vi "forced_vibration_and_shock.vi"() -> ()   [LabVIEW 2024]
uses:
  <vilib>/DAQmx/read.llb/DAQmx Read (Analog 1D Wfm NChan NSamp).vi
  <vilib>/DAQmx/create/channels.llb/DAQmx Create Channel (AI-Voltage-Basic).vi
  <vilib>/DAQmx/create/channels.llb/DAQmx Create Channel (AI-Acceleration-Accelerometer).vi
  <vilib>/DAQmx/configure/timing.llb/DAQmx Timing (Sample Clock).vi
  <vilib>/express/express analysis/Spectral/Block/exnSpectralBlock spectral measurements RMS poly.vi
  <vilib>/express/express analysis/Spectral/Block/exnSpectralBlock spectral measurements RMS WFM.vi
  <vilib>/express/express shared/transition.llb/Dynamic To Waveform Array.vi
  <vilib>/express/express signal manip/GetorSetDDTAttributes/Set DDT Attributes/SetT0.vi
  <vilib>/express/express shared/transition.llb/Waveform Array To Dynamic.vi
  <vilib>/DAQmx/miscellaneous.llb/DAQmx Fill In Error Info.vi
  <vilib>/express/express analysis/Spectral/Block/exnSpectralBlock spectral measurements RMS DDT.vi
  <vilib>/express/express analysis/Spectral/XNode/ExpressSpectralMeasurementsBlockNode.xnode
  <vilib>/express/express signal manip/GetorSetDDTAttributes/Set DDT Attributes/Set DDT Properties.xnode
  <resource>/objmgr/daqmx.rc
  <vilib>/measure/NI_MAPro.lvlib
panel:
  out "Waveform Graph 6":waveform(dbl)(graph)
  out "error out 4":errorcluster
  in  "error in (no error) 4":errorcluster
  in  "sampling info 3":cluster{"Fs":dbl, "#s":dbl}={"Fs"=1000.0, "#s"=1000.0} {"Fs" format="%.2p"}
  in  "frequency 3":dbl=10.0 format="%0.2p"
  in  "amplitude 3":dbl=1.0 format="%0.2p"
  in  "formula 3":string="sin(w*t)*sin(2*pi(1)*t)"
  out "Waveform Graph 5":waveform(dbl)(graph)
  out "Array":dbl[](array[numeric])
  in  "Numeric 2":dbl
  in  "Numeric 3":dbl
  in  "?":path
  out "Filename Out 3":path caption="Filename Out"
  out "AO_output_acc":waveform(dbl)(graph)
  out "AO_input_acc":waveform(dbl)(graph)
  out "AO_Voltage":waveform(dbl)(graph)
  out "FFT magnitude 3":dynamicdata(graph)
  out "ACC Time domain 3":dynamicdata(graph)
  out "VOLT Time domain 2":dynamicdata(graph)
  out "FFT magnitude 2":dynamicdata(graph)
  out "error out 2":errorcluster
  in  "error in (no error) 2":errorcluster
  in  "sampling info 2":cluster{"Fs":dbl, "#s":dbl}={"Fs"=1000.0, "#s"=1000.0} {"Fs" format="%.2p"}
  in  "frequency 2":dbl=10.0 format="%0.2p"
  in  "amplitude 2":dbl=1.0 format="%0.2p"
  in  "formula 2":string="sin(w*t)*sin(2*pi(1)*t)"
  out "Waveform Graph 4":waveform(dbl)(graph)
  out "error out":errorcluster
  in  "error in (no error)":errorcluster
  in  "sampling info":cluster{"Fs":dbl, "#s":dbl}={"Fs"=1000.0, "#s"=1000.0} {"Fs" format="%.2p"}
  in  "frequency":dbl=10.0 format="%0.2p"
  in  "amplitude":dbl=1.0 format="%0.2p"
  in  "formula":string="sin(w*t)*sin(2*pi(1)*t)"
  out "Waveform Graph 3":waveform(dbl)(graph)
  out "end index":i32
  out "start index":i32
  in  "end time":dbl
  in  "start time":dbl
  out "FFT excitation":cluster{"f0":dbl, "df":dbl, "magnitude":dbl[]}(graph)
  in  "voltage scale":dbl
  in  "output frequency":dbl
  # "frame_1"
  # "frame_3"
  # "0.1*sin(2*3.1416*5*t) + 2*exp(-((t-4)^2)/(2*0.05^2))"
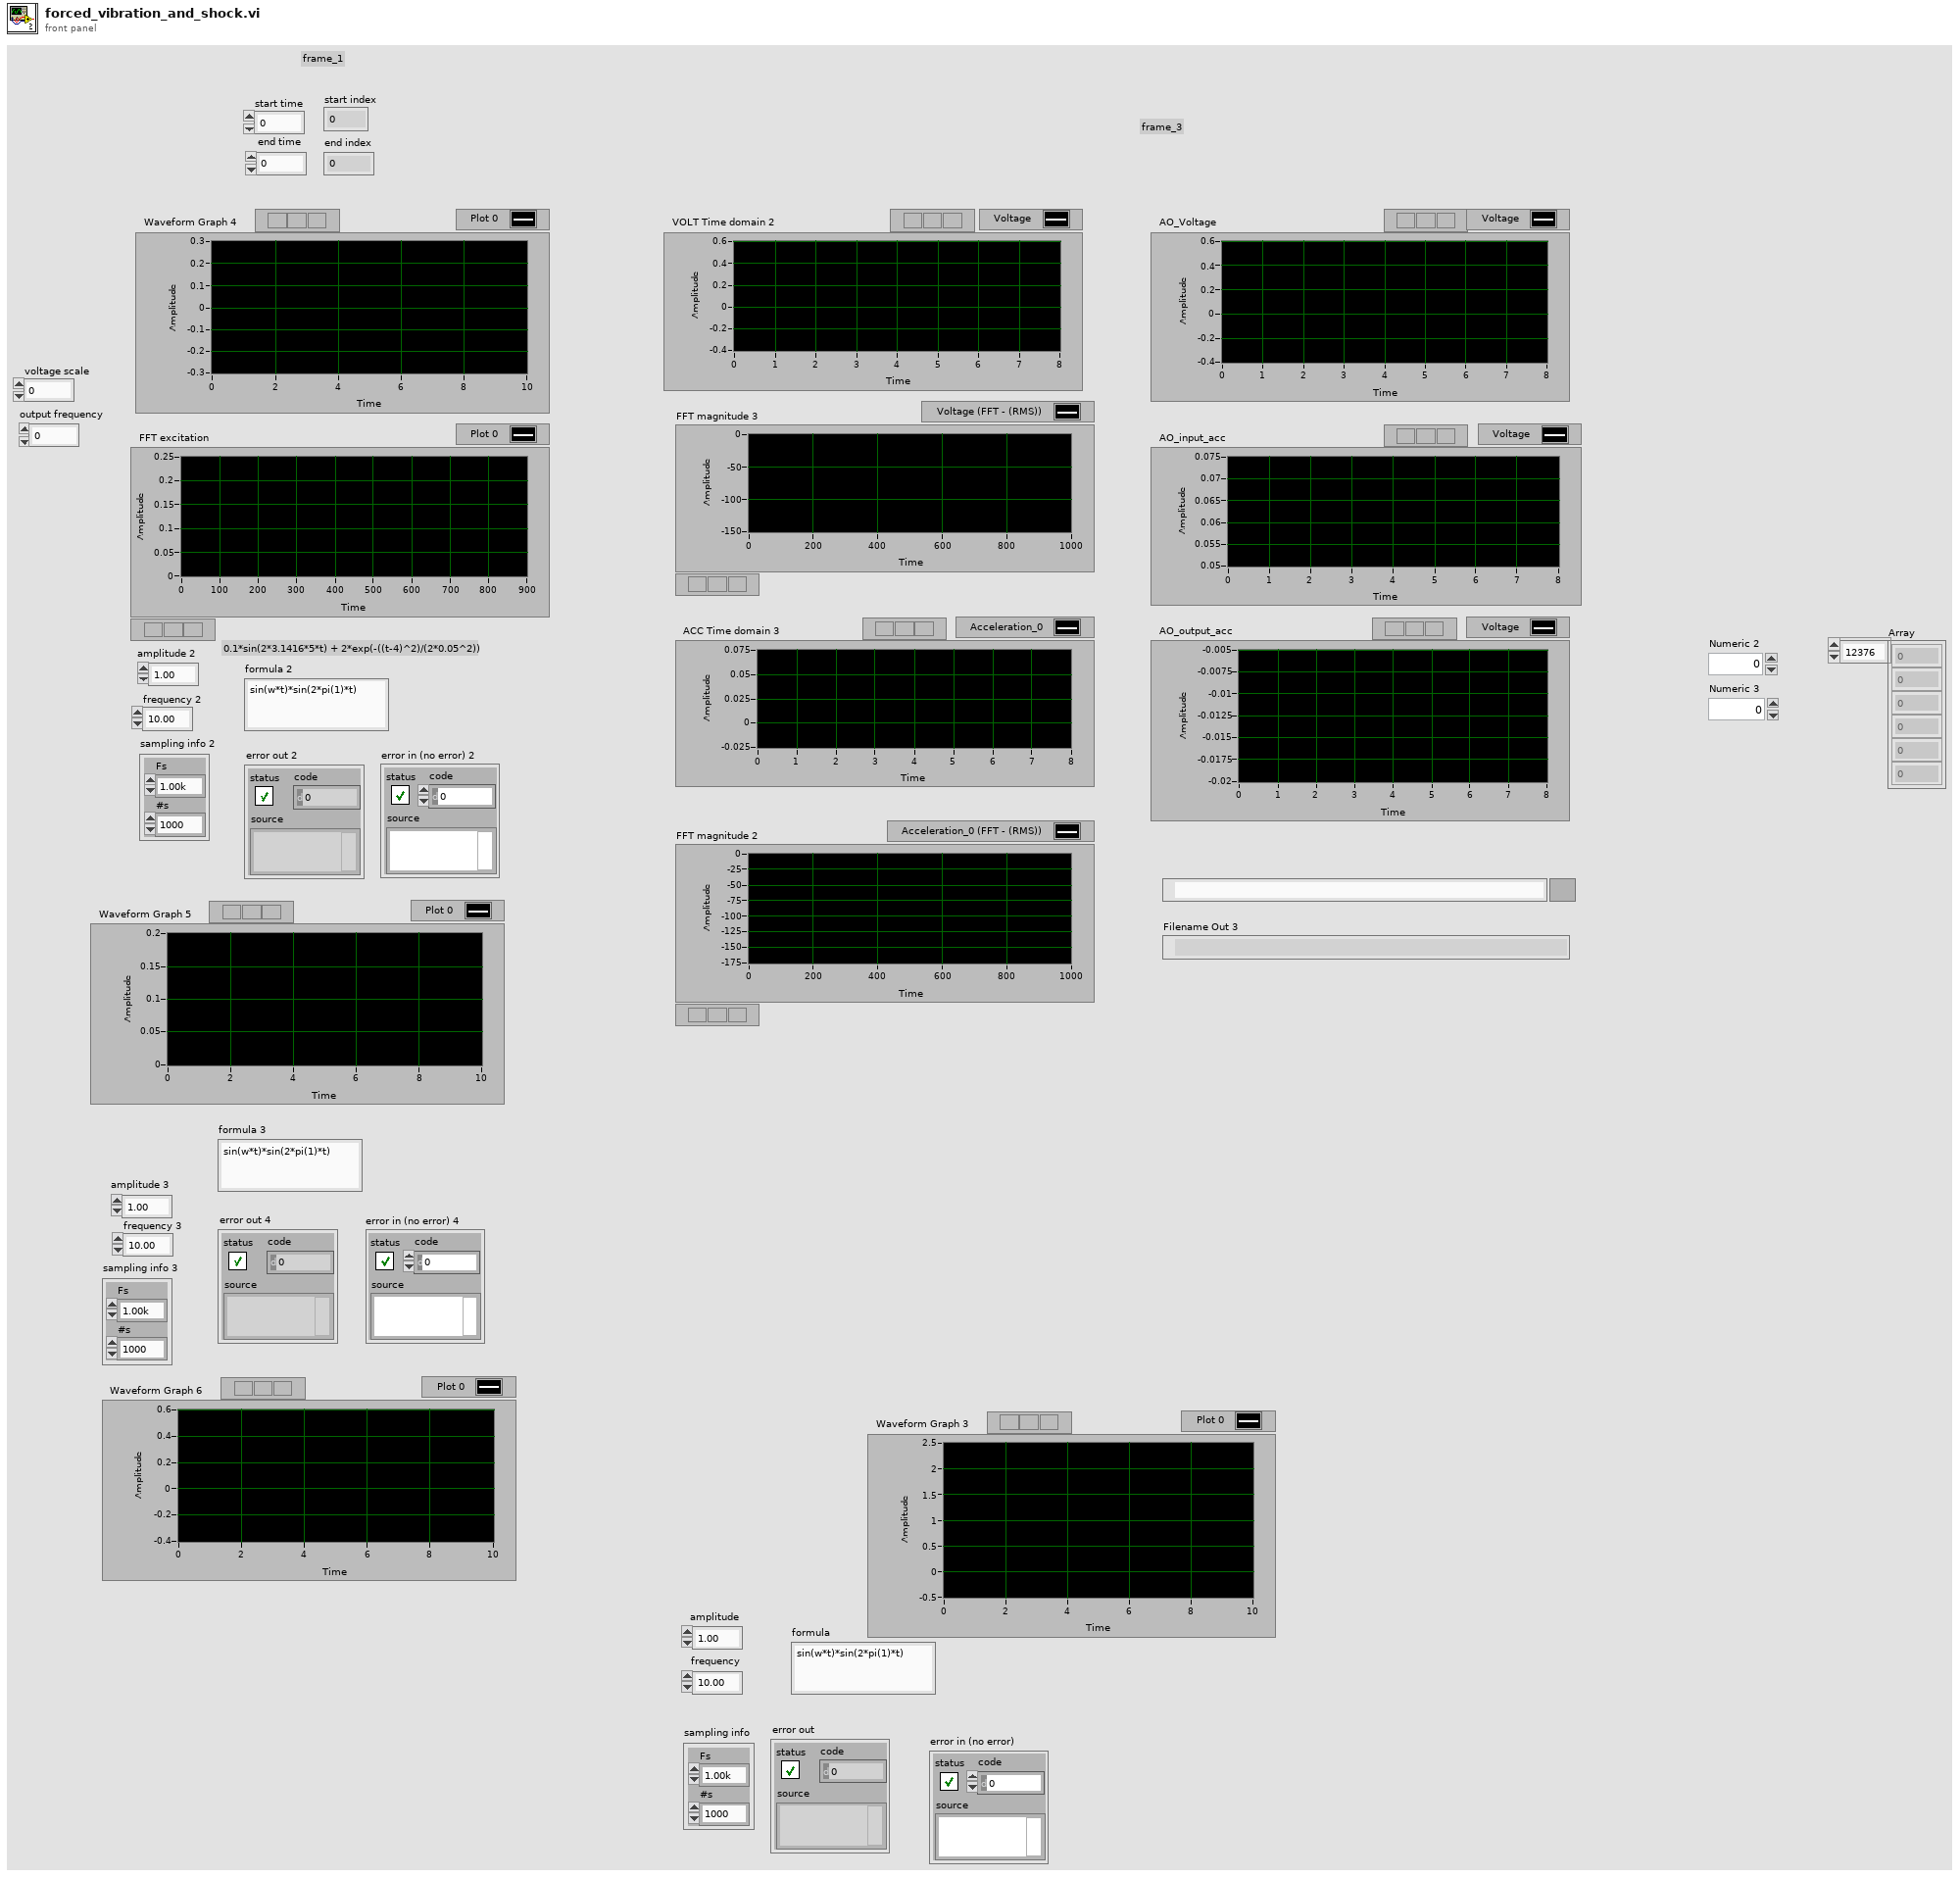
[diagram p1: front panel]
types:
  T1 = cluster{"averaging mode":u16, "weighting mode":u16, "number of averages":u32}
  T2 = cluster{"dB On (F)":bool, "unwrap phase (F)":bool, "convert to degree (F)":bool}
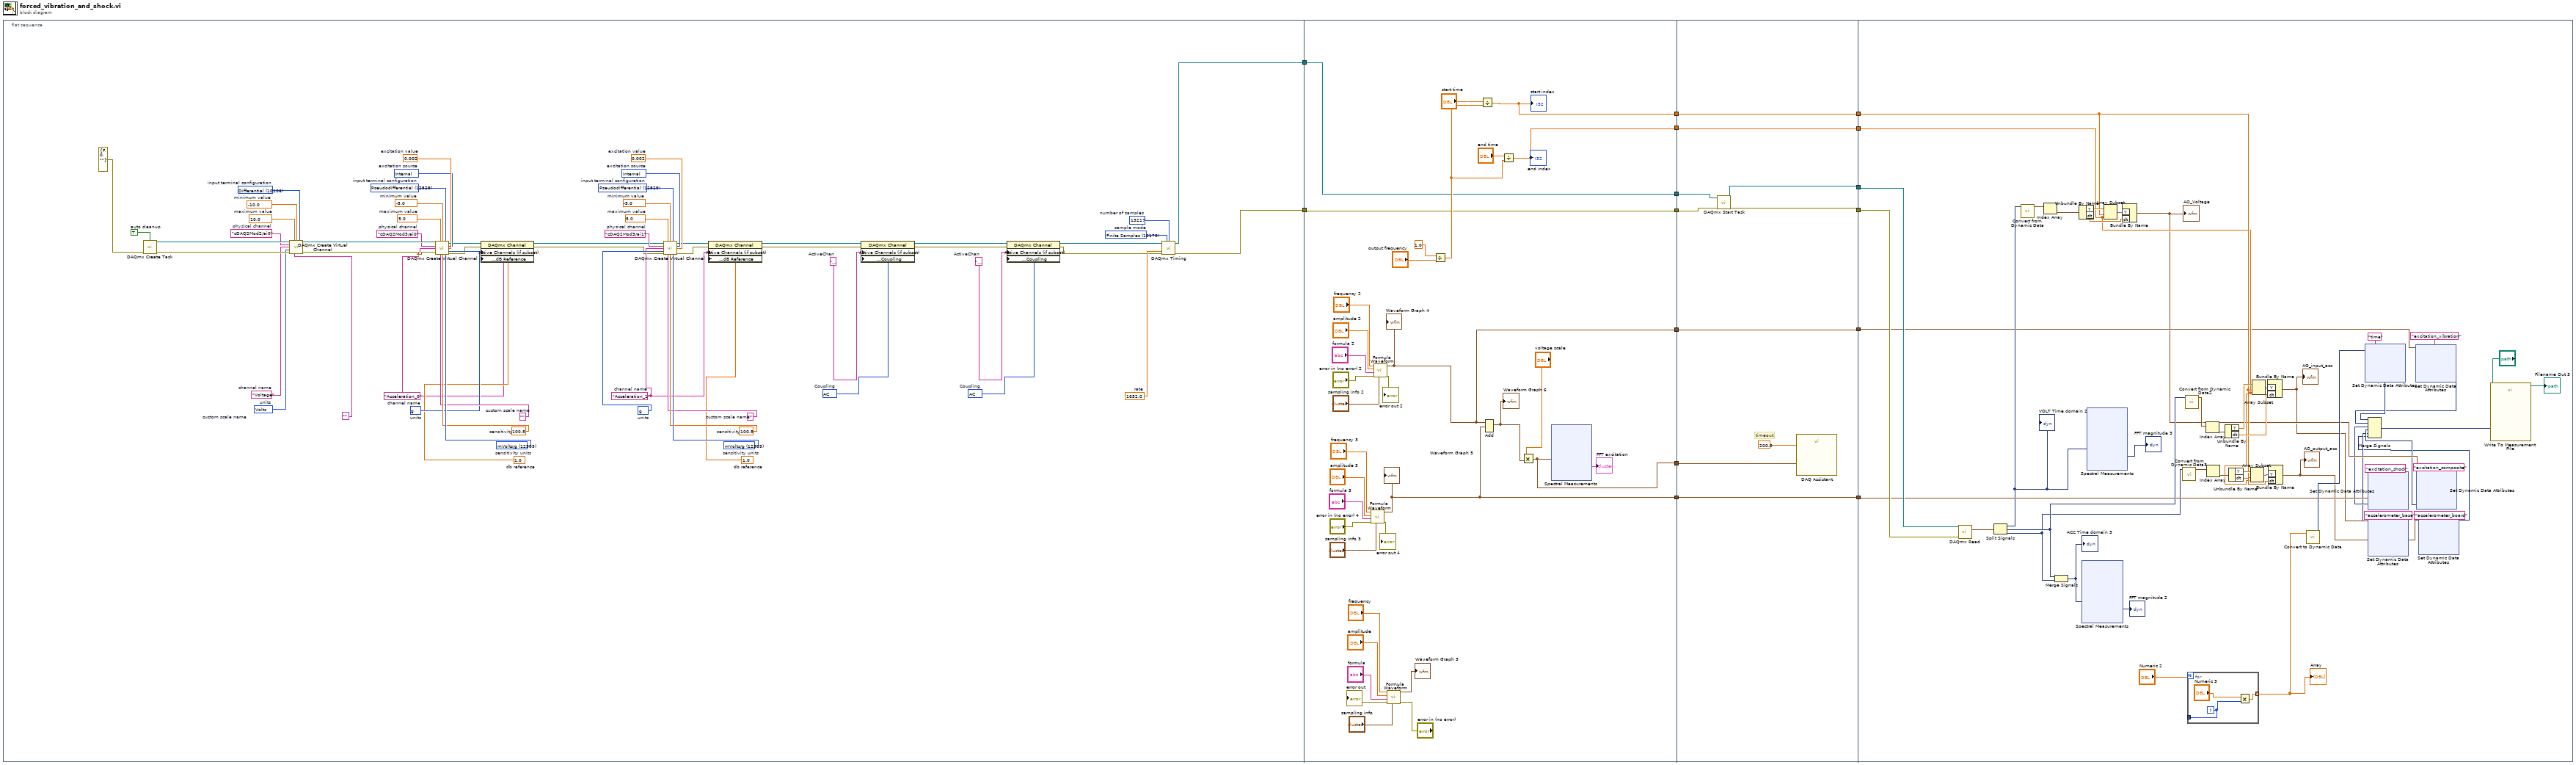
[diagram p0: block diagram]
diagram:
  n1 = flat-sequence {
    tunnel: [w17] -> w15
    tunnel: [w16] -> w11
    tunnel: w15 -> [w87]
    tunnel: [w76] -> w14
    tunnel: [w87] -> w13
    tunnel: [w86] -> w12
    tunnel: w11 -> [w86]
    tunnel: [w85] -> w7
    tunnel: [w84] -> w5
    tunnel: [w75] -> w3
    tunnel: [w74] -> w1
    tunnel: w14 -> [w126]
    tunnel: w13 -> [w125]
    tunnel: w12 -> [w124]
    tunnel: [w123] -> w10
    tunnel: [w122] -> w9
    tunnel: [w121] -> w8
    tunnel: w7 -> [w121]
    tunnel: [w120] -> w6
    tunnel: w5 -> [w120]
    tunnel: [w119] -> w4
    tunnel: w3 -> [w119]
    tunnel: [w118] -> w2
    tunnel: w1 -> [w118]
    tunnel: w10 -> [w149]
    tunnel: w9 -> [w148]
    tunnel: w8 -> [w151]
    tunnel: w6 -> [w150]
    tunnel: w4 -> [w141]
    tunnel: w2 -> [w140]
    frame #0 {
      w63 = 10106 items=["default"=-1, "RSE"=10083, "NRSE"=10078, "Differential"=10106, "Pseudodifferential"=12529]  # input terminal configuration
      w64 = 10348 items=["Volts"=10348, "From Custom Scale"=10065]  # units
      w65 = "Voltage"  # channel name
      w66 = ""  # custom scale name
      w67 = -10.0  # minimum value
      w68 = 10.0  # maximum value
      w69 = "cDAQ2Mod2/ai0"  # physical channel
      w30 = 10178 items=["Finite Samples"=10178, "Continuous Samples"=10123, "Hardware Timed Single Point"=12522]  # sample mode
      w31 = 13217  # number of samples
      w32 = 1652.0  # rate
      w34 = 10045 items=["AC"=10045, "DC"=10050, "GND"=10066]  # Coupling
      w33 = "Acceleration_1"  # ActiveChan
      w36 = 10045 items=["AC"=10045, "DC"=10050, "GND"=10066]  # Coupling
      w35 = "Acceleration_0"  # ActiveChan
      w38 = 1.0  # db reference
      w45 = 10186 items=["g"=10186, "m/s^2"=12470, "From Custom Scale"=10065]  # units
      w41 = 12529 items=["default"=-1, "RSE"=10083, "NRSE"=10078, "Differential"=10106, "Pseudodifferential"=12529]  # input terminal configuration
      w43 = 10200 items=["Internal"=10200, "External"=10167, "None"=10230]  # excitation source
      w44 = 0.002  # excitation value
      w48 = 12509 items=["mVolts/g"=12509, "Volts/g"=12510]  # sensitivity units
      w47 = 100.5  # sensitivity
      w37 = "Acceleration_1"  # channel name
      w46 = ""  # custom scale name
      w40 = -5.0  # minimum value
      w39 = 5.0  # maximum value
      w42 = "cDAQ2Mod3/ai1"  # physical channel
      w50 = 1.0  # db reference
      w57 = 10186 items=["g"=10186, "m/s^2"=12470, "From Custom Scale"=10065]  # units
      w53 = 12529 items=["default"=-1, "RSE"=10083, "NRSE"=10078, "Differential"=10106, "Pseudodifferential"=12529]  # input terminal configuration
      w55 = 10200 items=["Internal"=10200, "External"=10167, "None"=10230]  # excitation source
      w56 = 0.002  # excitation value
      w60 = 12509 items=["mVolts/g"=12509, "Volts/g"=12510]  # sensitivity units
      w59 = 100.5  # sensitivity
      w49 = "Acceleration_0"  # channel name
      w58 = ""  # custom scale name
      w52 = -5.0  # minimum value
      w51 = 5.0  # maximum value
      w54 = "cDAQ2Mod3/ai0"  # physical channel
      w61 = TRUE  # auto cleanup
      n2 = call <vilib>:"DAQmx Create Task.vi"("auto cleanup"=w61, "error in"=errorcluster {"status"=FALSE, "code"=0, "source"=""}) -> ("task out"=w70:refnum<k21>, "error out"=w71:errorcluster)  [unwired: 12 in]
      n3 = call-poly <vilib>:"DAQmx Create Virtual Channel.vi"("task in"=w70, "maximum value"=w68, "minimum value"=w67, "input terminal configuration"=w63, "physical channels"=w69, "name to assign"=w65, "units"=w64, "error in"=w71, "custom scale name"=w66) -> ("task out"=w72:refnum<k21>, "error out"=w73:errorcluster)  [unwired: 5 in]
      n4 = call-poly <vilib>:"DAQmx Create Virtual Channel.vi"("task in"=w72, "maximum value"=w51, "minimum value"=w52, "input terminal configuration"=w53, "physical channels"=w54, "current excitation source"=w55, "name to assign"=w49, "current excitation value"=w56, "units"=w57, "error in"=w73, "custom scale name"=w58, "sensitivity"=w59, "sensitivity units"=w60) -> ("task out"=w18:refnum<k21>, "error out"=w19:errorcluster)  [unwired: 1 in]
      n5 = property class="DAQmx Channel"(reference=w18, error in=w19, "Active Channels (if subset)"=w49, "Analog Input:Acceleration:dB Reference"=w50) -> (reference out=w21:refnum<k21>, error out=w20:errorcluster)
      n6 = call-poly <vilib>:"DAQmx Create Virtual Channel.vi"("task in"=w21, "maximum value"=w39, "minimum value"=w40, "input terminal configuration"=w41, "physical channels"=w42, "current excitation source"=w43, "name to assign"=w37, "current excitation value"=w44, "units"=w45, "error in"=w20, "custom scale name"=w46, "sensitivity"=w47, "sensitivity units"=w48) -> ("task out"=w22:refnum<k21>, "error out"=w23:errorcluster)  [unwired: 1 in]
      n7 = property class="DAQmx Channel"(reference=w22, error in=w23, "Active Channels (if subset)"=w37, "Analog Input:Acceleration:dB Reference"=w38) -> (reference out=w26:refnum<k21>, error out=w24:errorcluster)
      n8 = property class="DAQmx Channel"(reference=w26, error in=w24, "Active Channels (if subset)"=w35, "Analog Input:General Properties:Input Configuration:Coupling"=w36) -> (reference out=w28:refnum<k21>, error out=w25:errorcluster)
      n9 = property class="DAQmx Channel"(reference=w28, error in=w25, "Active Channels (if subset)"=w33, "Analog Input:General Properties:Input Configuration:Coupling"=w34) -> (reference out=w29:refnum<k21>, error out=w27:errorcluster)
      n10 = call-poly <vilib>:"DAQmx Timing.vi"("task/channels in"=w29, "sample mode"=w30, "samples per channel"=w31, "rate"=w32, "error in"=w27) -> ("task out"=w17:refnum<k21>, "error out"=w16:errorcluster)  [unwired: 9 in]
    }
    frame #1 {
      n11 = call <vilib>:"Formula Waveform.vi"("sampling info"="sampling info 3", "error in (no error)"="error in (no error) 4", "formula"="formula 3", "amplitude"="amplitude 3", "frequency"="frequency 3") -> ("error out"=→"error out 4":errorcluster, "signal out"=w74:waveform(dbl))  [unwired: 5 in]
      "Waveform Graph 5" <- w74
      n12 = call <vilib>:"Formula Waveform.vi"("sampling info"="sampling info 2", "error in (no error)"="error in (no error) 2", "formula"="formula 2", "amplitude"="amplitude 2", "frequency"="frequency 2") -> ("error out"=→"error out 2":errorcluster, "signal out"=w75:waveform(dbl))  [unwired: 5 in]
      "Waveform Graph 4" <- w75
      n13 = call <vilib>:"Formula Waveform.vi"("sampling info"="sampling info", "error in (no error)"="error in (no error)", "formula"="formula", "amplitude"="amplitude", "frequency"="frequency") -> ("error out"=→"error out":errorcluster, "signal out"=→"Waveform Graph 3":waveform(dbl))  [unwired: 5 in]
      n14 = Divide(x=1.0, y="output frequency") -> (x/y=w102:dbl)
      n15 = Divide(x="start time", y=w102) -> (x/y=w85:dbl)
      "start index" <- w85
      n16 = Add(1:w74, 2:w75) -> (0:w77:waveform(dbl))  [unwired: 1 in, 1 out]
      "Waveform Graph 6" <- w77
      n17 = Divide(x="end time", y=w102) -> (x/y=w84:dbl)
      "end index" <- w84
      n18 = Multiply(x="voltage scale", y=w77) -> (x*y=w76:waveform(dbl))
      n19 = xnode "Spectral Measurements"("Signals"=w76) -> ("FFT - (RMS)"=→"FFT excitation":cluster{"f0":dbl, "df":dbl, "magnitude":dbl[]})  [unwired: 1 in, 2 out]
    }
    frame #2 {
      # "timeout"
      n20 = call <vilib>:"DAQmx Start Task.vi"("task/channels in"=w125, "error in"=w124) -> ("task out"=w123:refnum<k21>, "error out"=w122:errorcluster)  [unwired: 12 in]
      n21 = call "DAQ Assistant"("data"=w126, "timeout (s)"=200.0) -> ()  [unwired: 16 in, 2 out]
    }
    frame #3 {
      n22 = call-poly <vilib>:"DAQmx Read.vi"("task/channels in"=w149, "error in"=w148) -> ("data"=w174:waveform(dbl)[])  [unwired: 11 in, 2 out]
      n23 = Split Signals(w174) -> (w173:dynamicdata, w156:dynamicdata, w155:dynamicdata)  [unwired: 3 in]
      "VOLT Time domain 2" <- w173
      n24 = call "Convert from Dynamic Data"("Dynamic Data Type"=w173) -> ("Array of Waveform"=w172:waveform(dbl)[])  [unwired: 3 in]
      n25 = Index Array(array=w172) -> (element=w171:waveform(dbl))  [unwired: 1 in]
      n26 = Merge Signals(w156, w155) -> (w154:dynamicdata)
      "ACC Time domain 3" <- w154
      n27 = Unbundle By Name(w171) -> ("Y"=w170:dbl[], "dt"=w169:dbl)
      n28 = xnode "Spectral Measurements"("Signals"=w154) -> ("FFT - (RMS)"=→"FFT magnitude 2":dynamicdata)  [unwired: 1 in, 2 out]
      n29 = xnode "Spectral Measurements"("Signals"=w173) -> ("FFT - (RMS)"=→"FFT magnitude 3":dynamicdata)  [unwired: 1 in, 2 out]
      n30 = Array Subset(array=w170, index=w151, length=w150) -> (w168:dbl[])
      n31 = Bundle By Name("Y"=w168, "dt"=w169) -> (w137:waveform(dbl))  [unwired: 1 in]
      "AO_Voltage" <- w137
      n32 = call "Convert from Dynamic Data3"("Dynamic Data Type"=w155) -> ("Array of Waveform"=w162:waveform(dbl)[])  [unwired: 3 in]
      n33 = call "Convert from Dynamic Data2"("Dynamic Data Type"=w156) -> ("Array of Waveform"=w167:waveform(dbl)[])  [unwired: 3 in]
      n34 = for {
        N: "Numeric 2" -> [_]
        tunnel: [w287] -> _
        tunnel: [w285] -> w147 mode=indexing
        i -> [w287]
        n35 = Multiply(x="Numeric 3", y=w287) -> (x*y=w285:dbl)
      }
      "Array" <- w147
      n36 = Index Array(array=w167) -> (element=w166:waveform(dbl))  [unwired: 1 in]
      n37 = Index Array(array=w162) -> (element=w161:waveform(dbl))  [unwired: 1 in]
      n38 = Unbundle By Name(w166) -> ("Y"=w165:dbl[], "dt"=w164:dbl)
      n39 = Unbundle By Name(w161) -> ("Y"=w160:dbl[], "dt"=w153:dbl)
      n40 = Array Subset(array=w160, index=w151, length=w150) -> (w159:dbl[])
      n41 = Array Subset(array=w165, index=w151, length=w150) -> (w163:dbl[])
      n42 = Bundle By Name("Y"=w163, "dt"=w164) -> (w136:waveform(dbl))  [unwired: 1 in]
      "AO_input_acc" <- w136
      n43 = Bundle By Name("Y"=w159, "dt"=w153) -> (w134:waveform(dbl))  [unwired: 1 in]
      "AO_output_acc" <- w134
      n44 = call "Convert to Dynamic Data"("Array"=w147) -> ("Dynamic Data Type"=w145:dynamicdata)  [unwired: 3 in]
      n45 = xnode "Set Dynamic Data Attributes"("Signals In"=w145, "Signal Name"="time") -> ("Signals Out"=w144:dynamicdata)  [unwired: 3 in, 1 out]
      n46 = xnode "Set Dynamic Data Attributes"("Signals In"=w136, "Signal Name"="accelerometer_base") -> ("Signals Out"=w129:dynamicdata)  [unwired: 3 in, 1 out]
      n47 = xnode "Set Dynamic Data Attributes"("Signals In"=w140, "Signal Name"="excitation_shock") -> ("Signals Out"=w131:dynamicdata)  [unwired: 3 in, 1 out]
      n48 = xnode "Set Dynamic Data Attributes"("Signals In"=w141, "Signal Name"="excitation_vibration") -> ("Signals Out"=w132:dynamicdata)  [unwired: 3 in, 1 out]
      n49 = xnode "Set Dynamic Data Attributes"("Signals In"=w137, "Signal Name"="excitation_composite") -> ("Signals Out"=w130:dynamicdata)  [unwired: 3 in, 1 out]
      n50 = xnode "Set Dynamic Data Attributes"("Signals In"=w134, "Signal Name"="accelerometer_board") -> ("Signals Out"=w128:dynamicdata)  [unwired: 3 in, 1 out]
      n51 = Merge Signals(w144, w132, w131, w130, w129, w128) -> (w146:dynamicdata)
      n52 = call "Write To Measurement File"("Signals"=w146, "Filename"="?") -> ("Filename Out"=→"Filename Out 3":path)  [unwired: 15 in, 2 out]
    }
  }
